vi "String to Enum.vi"(8 "error in":errorcluster, 11 "string in":string) -> (0 "error out":errorcluster, 3 "enum out":T1)   [LabVIEW 2018]
uses:
  Type Defs/SR Status.ctl
panel:
  out "SR Status":T1
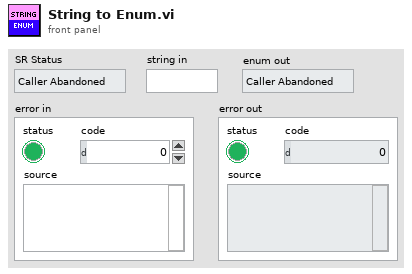
[diagram p1: front panel]
types:
  T1 = typedef "SR Status.ctl" = enum16{"Caller Abandoned", "Created in Error", "Expired", "Forum Resolved AE", "Forum Resolved Customer", "IN WORK", "IN WORK Collab with AES", "IN WORK Collab with PSE", "IN WORK Collab with SE", "IN WORK Customer Added Note", "IN WORK Escalation", "IN WORK Wait on Customer", "Open", "Potentially Resolved", "Presumed Resolved", "RMA Approved for Return", "Resolved", "Passed Off"}
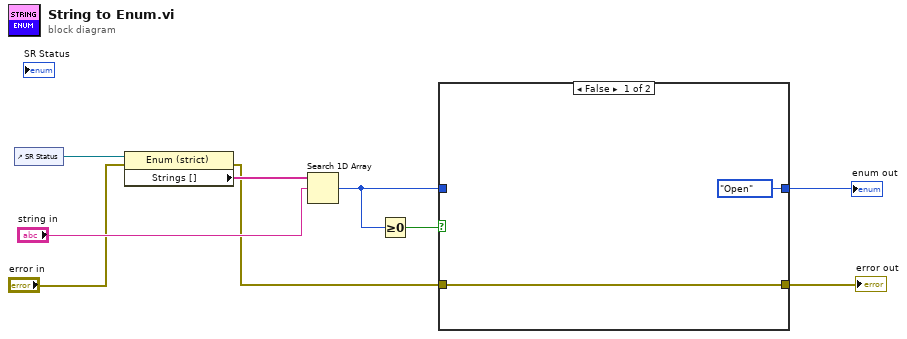
[diagram p0: block diagram]
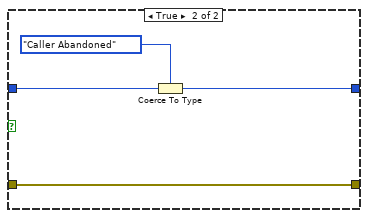
[diagram p2: hidden frame]
diagram:
  n1 = control-ref of="SR Status"() -> (w9:refnum<vi>)
  n2 = property class="Enum (strict)"(reference=w9, error in="error in") -> (error out=w2:errorcluster, "Strings []"=w8:string[])  [unwired: 1 out]
  n3 = Search 1D Array(1D array=w8, element="string in") -> (index of element=w6:i32)  [unwired: 1 in]
  n4 = Greater Or Equal To 0?(x=w6) -> (x >= 0?=w7:bool)
  n5 = case shown="False" w7 {
    tunnel: w6 -> [_ w15]
    tunnel: [SR_Status."Open" ("SR Status 2") w13] -> w4
    tunnel: w2 -> [w11 w12]
    tunnel: [w11 w12] -> w1
    frame False {
    }
    frame True {
      n6 = Coerce To Type(0:w15, 1:SR_Status."Caller Abandoned" ("SR Status 2")) -> (2:w13:T1)
    }
  }
  "enum out" <- w4
  "error out" <- w1
